vi "hydrolyse_reactor.vi"(2 "#":i16, 4 "Dataflow In":errorcluster) -> (1 "Dataflow Out":errorcluster)   [LabVIEW 2019]
uses:
  lib/libSimulationControl/libSimulationControl.lvlib
panel:
  # "*******************************************************************\nBiogas Plant Control\n\nAuthor: Paul Zügel\nGCSC-Frankfurt am Main 2020\n\n*******************************************************************"
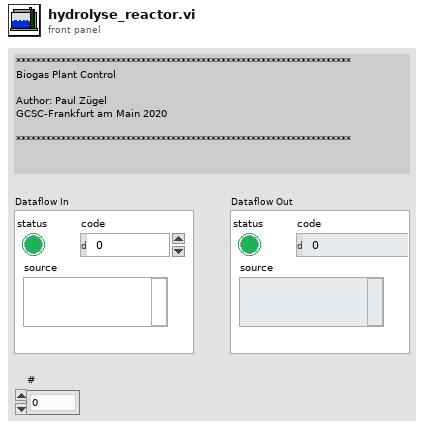
[diagram p1: front panel]
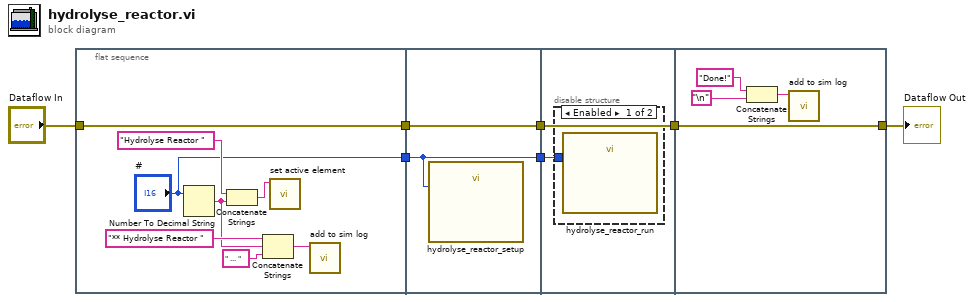
[diagram p0: block diagram]
diagram:
  n1 = flat-sequence {
    tunnel: "Dataflow In" -> [w15]
    tunnel: [w15] -> w6
    tunnel: ["#"] -> w4
    tunnel: [w17] -> w3
    tunnel: w6 -> [w17]
    tunnel: w4 -> [w16]
    tunnel: [w16] -> w1
    tunnel: w3 -> [w19]
    tunnel: [w19] -> w2
    tunnel: w1 -> [w18]
    tunnel: [w24] -> w5
    tunnel: w2 -> [w24]
    frame #0 {
      n2 = Number To Decimal String(number="#") -> (decimal integer string=w11:string)  [unwired: 1 in]
      n3 = Concatenate Strings("Hydrolyse Reactor " ("elem"), w11) -> (w13:string)
      n4 = Concatenate Strings("** Hydrolyse Reactor " ("string"), w11, " ... " ("string")) -> (w9:string)
      n5 = call "set active element.vi"("elem"=w13) -> ()  [unwired: 10 in, 1 out]
      n6 = call "add to sim log.vi"("log"=w9) -> ()  [unwired: 10 in, 1 out]
    }
    frame #1 {
      n7 = call "hydrolyse_reactor_setup.vi"("#"=w16) -> ()  [unwired: 11 in]
    }
    frame #2 {
      n8 = disable-structure shown="Enabled" {
        disable-tunnel: w18 -> [w20 _]
        frame Enabled {
          n9 = call "hydrolyse_reactor_run.vi"("#"=w20) -> ()  [unwired: 11 in]
        }
        frame Disabled {
        }
      }
    }
    frame #3 {
      n10 = Concatenate Strings("Done!" ("string"), "\n") -> (w21:string)
      n11 = call "add to sim log.vi"("log"=w21) -> ()  [unwired: 10 in, 1 out]
    }
  }
  "Dataflow Out" <- w5
